vi "Estrazione Energia Detector.vi"(6 "External File?":bool, 7 "file path (dialog if empty)":path, 11 "Detector In":dbl[][](array[numeric])) -> (3 "detector-lines":T1)   [LabVIEW 2023]
uses:
  <vilib>/Utility/file.llb/Read Delimited Spreadsheet (DBL).vi
  <vilib>/gmath/NI_Gmath.lvlib
panel:
  out "Detector":dbl[][](array[numeric])
  out "Array":dbl[][](array[numeric])
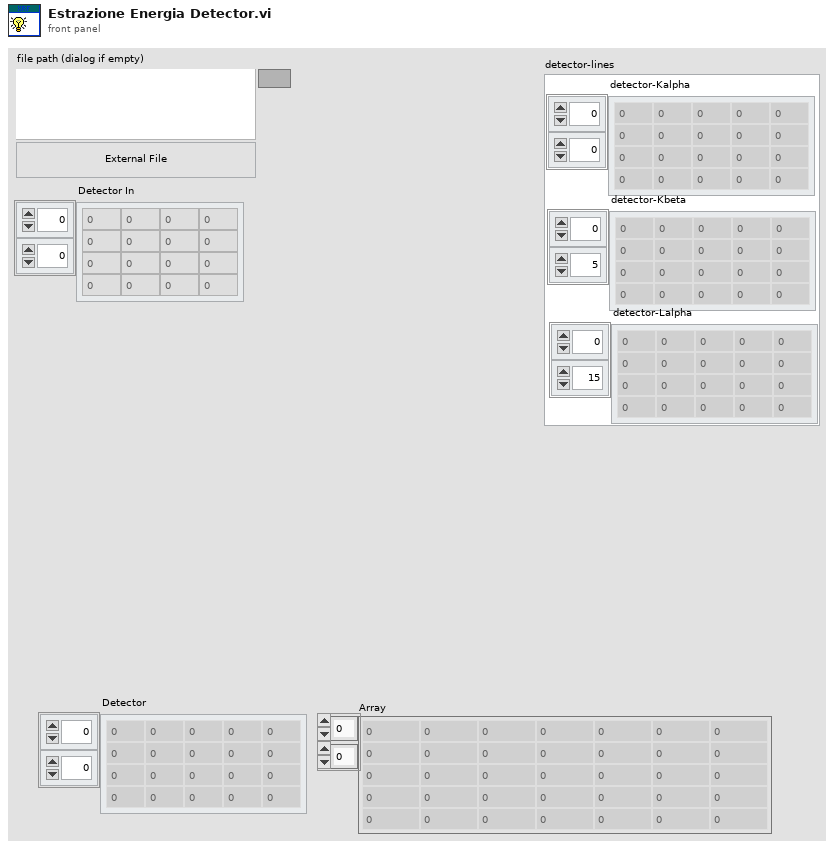
[diagram p1: front panel]
types:
  T1 = cluster{"detector-Kalpha":dbl[][], "detector-Kbeta":dbl[][], "detector-Lalpha":dbl[][]}
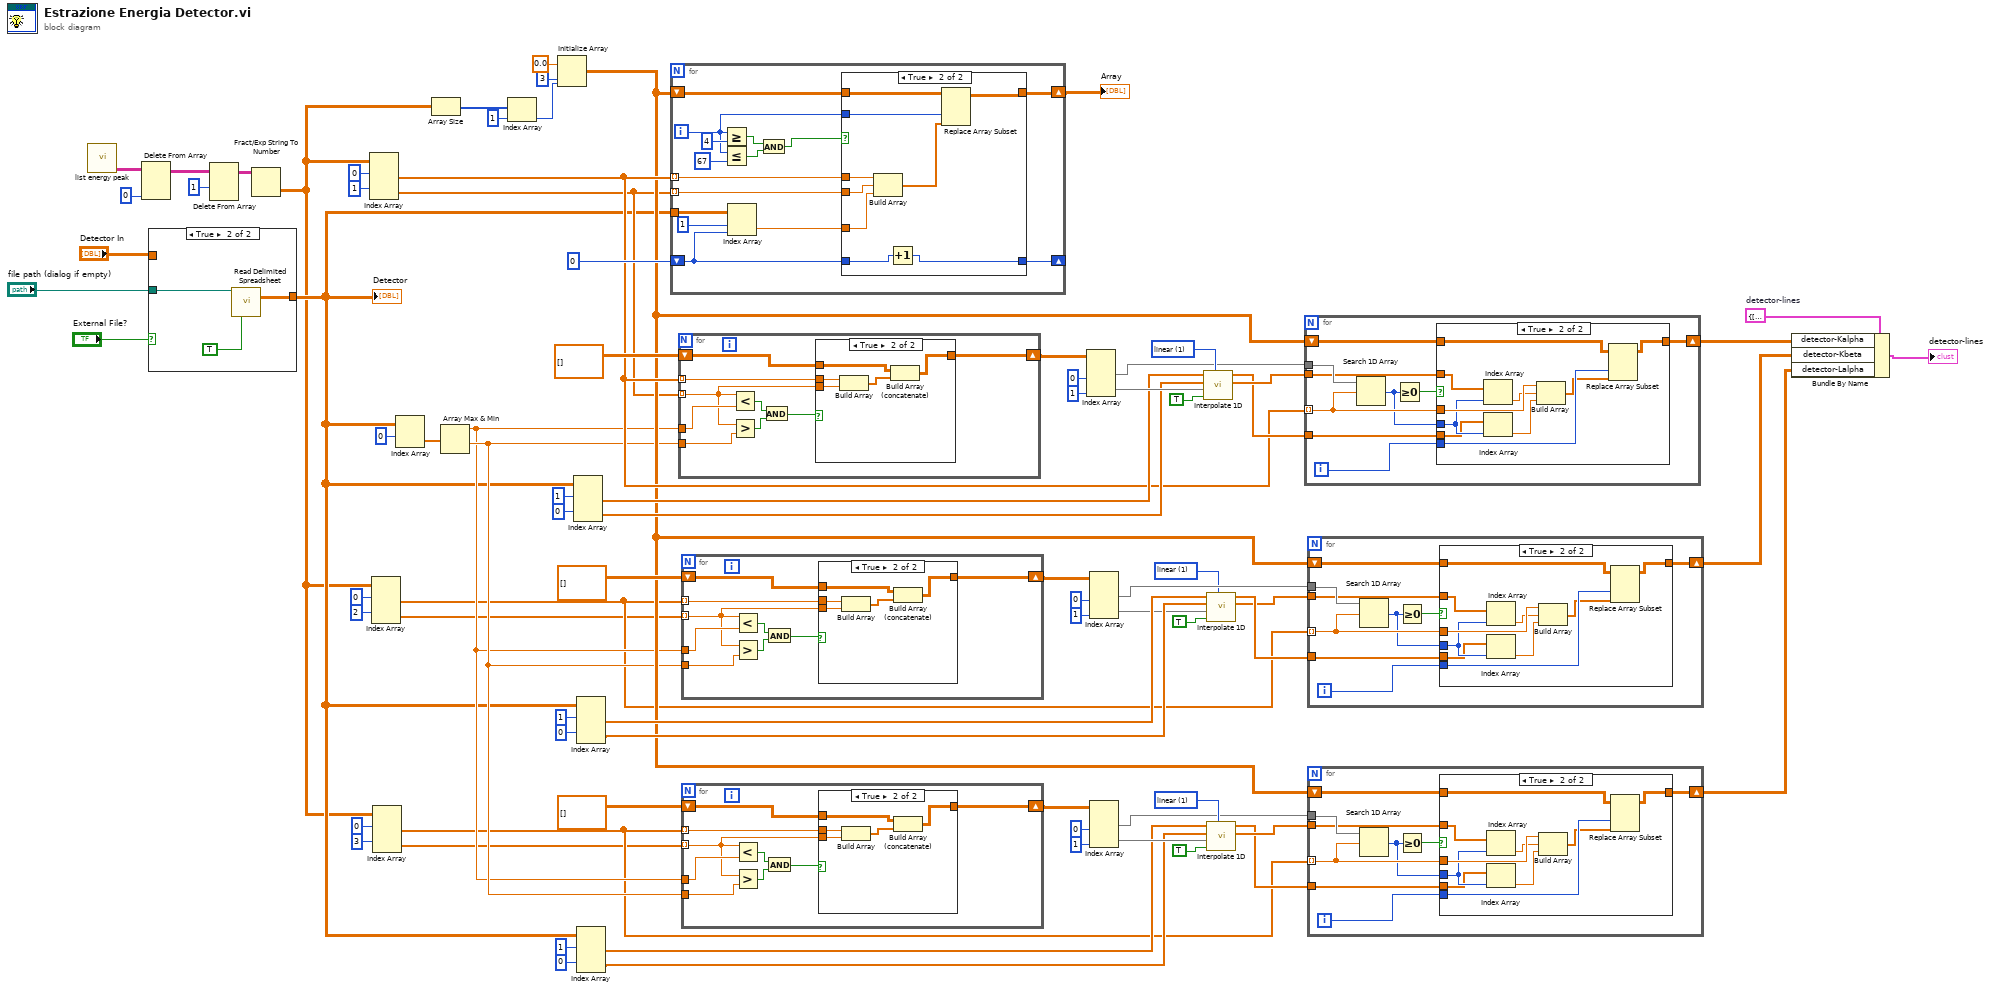
[diagram p0: block diagram]
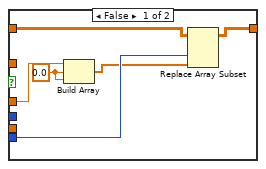
[diagram p2: hidden frame]
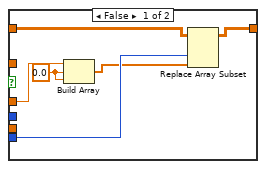
[diagram p4: hidden frame]
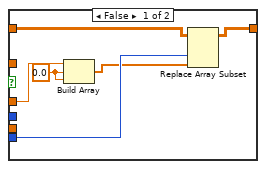
[diagram p6: hidden frame]
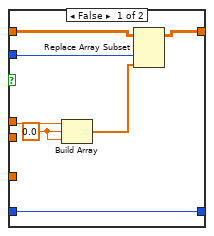
[diagram p8: hidden frame]
diagram:
  w14 = T1 {"detector-Kalpha"=[], "detector-Kbeta"=[], "detector-Lalpha"=[]}  # detector-lines
  w31 = 1 items=["nearest", "linear", "spline", "cubic Hermite", "Lagrange"] ("method")
  w40 = 1 items=["nearest", "linear", "spline", "cubic Hermite", "Lagrange"] ("method")
  w61 = 1 items=["nearest", "linear", "spline", "cubic Hermite", "Lagrange"] ("method")
  n1 = call "list energy peak.vi"() -> ("Lines"=w77:string[][])  [unwired: 6 in, 5 out]
  n2 = Delete From Array(array=w77, index (col)=0 ("disabled index (col)")) -> (array with subset deleted=w79:string[][])  [unwired: 2 in, 1 out]
  n3 = case shown="True" "External File?" {
    tunnel: [w82 w84] -> w15
    tunnel: "file path (dialog if empty)" -> [_ w83]
    tunnel: "Detector In" -> [w82 _]
    frame False {
    }
    frame True {
      n4 = call-poly <vilib>:"Read Delimited Spreadsheet.vi"("file path (dialog if empty)"=w83, "transpose? (F)"=TRUE) -> ("all rows"=w84:dbl[][])  [unwired: 8 in, 5 out]
    }
  }
  "Detector" <- w15
  n5 = Delete From Array(array=w79, index (row)=1 ("disabled index (col)")) -> (array with subset deleted=w78:string[][])  [unwired: 2 in, 1 out]
  n6 = Fract/Exp String To Number(string=w78) -> (number=w1:dbl[][])  [unwired: 3 in, 1 out]
  n7 = Index Array(array=w1, index (row) #1=0 ("index (row)"), index (row) #2=1 ("index (row)")) -> (element #1=w20:dbl[], element #2=w16:dbl[])  [unwired: 2 in]
  n8 = Index Array(array=w1, index (row) #1=0 ("index (row)"), index (row) #2=2 ("index (row)")) -> (element #1=w5:dbl[], element #2=w4:dbl[])  [unwired: 2 in]
  n9 = Index Array(array=w1, index (row) #1=0 ("index (row)"), index (row) #2=3 ("index (row)")) -> (element #1=w3:dbl[], element #2=w2:dbl[])  [unwired: 2 in]
  n10 = Index Array(array=w15, index (row)=0) -> (element=w66:dbl[])  [unwired: 1 in]
  n11 = Array Size(array=w1) -> (size(s)=w72:i32[])
  n12 = Array Max & Min(array=w66) -> (max value=w17:dbl, min value=w18:dbl)  [unwired: 2 out]
  n13 = Index Array(array=w72, index=1) -> (element=w67:i32)
  n14 = Initialize Array(0.0 ("element"), 3 ("dimension size"), w67) -> (w19:dbl[][])
  n15 = Index Array(array=w15, index (row) #1=1 ("index (row)"), index (row) #2=0 ("index (row)")) -> (element #1=w54:dbl[], element #2=w53:dbl[])  [unwired: 2 in]
  n16 = Index Array(array=w15, index (row) #1=1 ("index (row)"), index (row) #2=0 ("index (row)")) -> (element #1=w47:dbl[], element #2=w48:dbl[])  [unwired: 2 in]
  n17 = Index Array(array=w15, index (row) #1=1 ("index (row)"), index (row) #2=0 ("index (row)")) -> (element #1=w24:dbl[], element #2=w23:dbl[])  [unwired: 2 in]
  n18 = for {
    tunnel: w20 -> [w91] mode=indexing
    tunnel: w16 -> [w92] mode=indexing
    tunnel: w15 -> [w100]
    shift-right: [w90] -> w36
    shift-left: w19 -> [w89]
    shift-right: [w86] -> _
    shift-left: 0 ("index (row)") -> [w87]
    i -> [w88]
    n19 = Greater Or Equal?(x=w88, y=4) -> (x >= y?=w96:bool)
    n20 = Less Or Equal?(x=w88, y=67) -> (x <= y?=w95:bool)
    n21 = Index Array(array=w100, index (row)=1 ("disabled index (col)"), index (col)=w87) -> (element=w93:dbl)
    n22 = And(x=w96, y=w95) -> (x .and. y?=w94:bool)
    n23 = case shown="True" w94 {
      tunnel: w93 -> [_ w111]
      tunnel: w92 -> [_ w112]
      tunnel: w91 -> [w105 w113]
      tunnel: [w102 w114] -> w90
      tunnel: w89 -> [w103 w116]
      tunnel: w88 -> [w106 w115]
      tunnel: w87 -> [w101 w109]
      tunnel: [w101 w108] -> w86
      frame False {
        w104 = 0.0
        n24 = Build Array(w105, w104, w104) -> (w107:dbl[])
        n25 = Replace Array Subset(array=w103, new element=w107, index (col)=w106) -> (w102:dbl[][])  [unwired: 1 in]
      }
      frame True {
        n26 = Build Array(w113, w112, w111) -> (w110:dbl[])
        n27 = Increment(x=w109) -> (x+1=w108:i32)
        n28 = Replace Array Subset(array=w116, new element=w110, index (col)=w115) -> (w114:dbl[][])  [unwired: 1 in]
      }
    }
  }
  "Array" <- w36
  n29 = for {
    shift-right: [w117] -> w59
    shift-left: dbl[][] [] -> [w120]
    tunnel: w20 -> [w119] mode=indexing
    tunnel: w16 -> [w118] mode=indexing
    tunnel: w17 -> [w123]
    tunnel: w18 -> [w122]
    n30 = Less?(x=w118, y=w123) -> (x < y?=w125:bool)
    n31 = Greater?(x=w118, y=w122) -> (0:w124:bool)
    n32 = And(x=w125, y=w124) -> (x .and. y?=w121:bool)
    n33 = case shown="True" w121 {
      tunnel: w120 -> [w126 w127]
      tunnel: w119 -> [_ w131]
      tunnel: w118 -> [_ w130]
      tunnel: [w126 w128] -> w117
      frame False {
      }
      frame True {
        n34 = Build Array(w131, w130) -> (w129:dbl[])
        n35 = Build Array (concatenate)(w127, w129) -> (w128:dbl[][])
      }
    }
  }
  n36 = for {
    shift-right: [w132] -> w42
    shift-left: dbl[][] [] -> [w135]
    tunnel: w5 -> [w134] mode=indexing
    tunnel: w4 -> [w133] mode=indexing
    tunnel: w17 -> [w138]
    tunnel: w18 -> [w137]
    n37 = Less?(x=w133, y=w138) -> (x < y?=w140:bool)
    n38 = Greater?(x=w133, y=w137) -> (0:w139:bool)
    n39 = And(x=w140, y=w139) -> (x .and. y?=w136:bool)
    n40 = case shown="True" w136 {
      tunnel: w135 -> [w141 w142]
      tunnel: w134 -> [_ w146]
      tunnel: w133 -> [_ w145]
      tunnel: [w141 w143] -> w132
      frame False {
      }
      frame True {
        n41 = Build Array(w146, w145) -> (w144:dbl[])
        n42 = Build Array (concatenate)(w142, w144) -> (w143:dbl[][])
      }
    }
  }
  n43 = for {
    shift-right: [w147] -> w29
    shift-left: dbl[][] [] -> [w150]
    tunnel: w3 -> [w149] mode=indexing
    tunnel: w2 -> [w148] mode=indexing
    tunnel: w17 -> [w153]
    tunnel: w18 -> [w152]
    n44 = Less?(x=w148, y=w153) -> (x < y?=w155:bool)
    n45 = Greater?(x=w148, y=w152) -> (0:w154:bool)
    n46 = And(x=w155, y=w154) -> (x .and. y?=w151:bool)
    n47 = case shown="True" w151 {
      tunnel: w150 -> [w156 w157]
      tunnel: w149 -> [_ w161]
      tunnel: w148 -> [_ w160]
      tunnel: [w156 w158] -> w147
      frame False {
      }
      frame True {
        n48 = Build Array(w161, w160) -> (w159:dbl[])
        n49 = Build Array (concatenate)(w157, w159) -> (w158:dbl[][])
      }
    }
  }
  n50 = Index Array(array=w59, index (col) #1=0 ("disabled index (col)"), index (col) #2=1 ("index (col)")) -> (element #1=w58:dbl[], element #2=w60:dbl[])  [unwired: 2 in]
  n51 = Index Array(array=w42, index (col) #1=0 ("disabled index (col)"), index (col) #2=1 ("index (col)")) -> (element #1=w43:dbl[], element #2=w41:dbl[])  [unwired: 2 in]
  n52 = Index Array(array=w29, index (col) #1=0 ("disabled index (col)"), index (col) #2=1 ("index (col)")) -> (element #1=w28:dbl[], element #2=w30:dbl[])  [unwired: 2 in]
  n53 = call <vilib>:"Interpolate 1D.vi"("method"=w61, "X is monotonic"=TRUE, "xi"=w60, "X"=w53, "Y"=w54) -> ("xi used"=w57:dbl[], "yi"=w51:dbl[])  [unwired: 4 in, 1 out]
  n54 = call <vilib>:"Interpolate 1D.vi"("method"=w40, "X is monotonic"=TRUE, "xi"=w41, "X"=w48, "Y"=w47) -> ("xi used"=w44:dbl[], "yi"=w50:dbl[])  [unwired: 4 in, 1 out]
  n55 = call <vilib>:"Interpolate 1D.vi"("method"=w31, "X is monotonic"=TRUE, "xi"=w30, "X"=w23, "Y"=w24) -> ("xi used"=w27:dbl[], "yi"=w21:dbl[])  [unwired: 4 in, 1 out]
  n56 = for {
    tunnel: w57 -> [w163]
    tunnel: w58 -> [w165]
    tunnel: w20 -> [w166] mode=indexing
    shift-right: [w169] -> w13
    shift-left: w19 -> [w170]
    tunnel: w51 -> [w162]
    i -> [w168]
    n57 = Search 1D Array(1D array=w165, element=w166) -> (index of element=w164:i32)  [unwired: 1 in]
    n58 = Greater Or Equal To 0?(x=w164) -> (x >= 0?=w167:bool)
    n59 = case shown="True" w167 {
      tunnel: w170 -> [w176 w186]
      tunnel: [w175 w185] -> w169
      tunnel: w168 -> [w174 w184]
      tunnel: w166 -> [w172 w183]
      tunnel: w164 -> [_ w182]
      tunnel: w163 -> [_ w181]
      tunnel: w162 -> [_ w178]
      frame False {
        w173 = 0.0
        n60 = Build Array(w172, w173, w173) -> (w171:dbl[])
        n61 = Replace Array Subset(array=w176, new element=w171, index (col)=w174) -> (w175:dbl[][])  [unwired: 1 in]
      }
      frame True {
        n62 = Index Array(array=w181, index=w182) -> (element=w179:dbl)
        n63 = Index Array(array=w178, index=w182) -> (element=w177:dbl)
        n64 = Build Array(w183, w179, w177) -> (w180:dbl[])
        n65 = Replace Array Subset(array=w186, new element=w180, index (col)=w184) -> (w185:dbl[][])  [unwired: 1 in]
      }
    }
  }
  n66 = for {
    tunnel: w44 -> [w188]
    tunnel: w43 -> [w190]
    tunnel: w5 -> [w191] mode=indexing
    shift-right: [w194] -> w12
    shift-left: w19 -> [w195]
    tunnel: w50 -> [w187]
    i -> [w193]
    n67 = Search 1D Array(1D array=w190, element=w191) -> (index of element=w189:i32)  [unwired: 1 in]
    n68 = Greater Or Equal To 0?(x=w189) -> (x >= 0?=w192:bool)
    n69 = case shown="True" w192 {
      tunnel: w195 -> [w201 w211]
      tunnel: [w200 w210] -> w194
      tunnel: w193 -> [w199 w209]
      tunnel: w191 -> [w197 w208]
      tunnel: w189 -> [_ w207]
      tunnel: w188 -> [_ w206]
      tunnel: w187 -> [_ w203]
      frame False {
        w198 = 0.0
        n70 = Build Array(w197, w198, w198) -> (w196:dbl[])
        n71 = Replace Array Subset(array=w201, new element=w196, index (col)=w199) -> (w200:dbl[][])  [unwired: 1 in]
      }
      frame True {
        n72 = Index Array(array=w206, index=w207) -> (element=w204:dbl)
        n73 = Index Array(array=w203, index=w207) -> (element=w202:dbl)
        n74 = Build Array(w208, w204, w202) -> (w205:dbl[])
        n75 = Replace Array Subset(array=w211, new element=w205, index (col)=w209) -> (w210:dbl[][])  [unwired: 1 in]
      }
    }
  }
  n76 = for {
    tunnel: w27 -> [w213]
    tunnel: w28 -> [w215]
    tunnel: w3 -> [w216] mode=indexing
    shift-right: [w219] -> w11
    shift-left: w19 -> [w220]
    tunnel: w21 -> [w212]
    i -> [w218]
    n77 = Search 1D Array(1D array=w215, element=w216) -> (index of element=w214:i32)  [unwired: 1 in]
    n78 = Greater Or Equal To 0?(x=w214) -> (x >= 0?=w217:bool)
    n79 = case shown="True" w217 {
      tunnel: w220 -> [w226 w236]
      tunnel: [w225 w235] -> w219
      tunnel: w218 -> [w224 w234]
      tunnel: w216 -> [w222 w233]
      tunnel: w214 -> [_ w232]
      tunnel: w213 -> [_ w231]
      tunnel: w212 -> [_ w228]
      frame False {
        w223 = 0.0
        n80 = Build Array(w222, w223, w223) -> (w221:dbl[])
        n81 = Replace Array Subset(array=w226, new element=w221, index (col)=w224) -> (w225:dbl[][])  [unwired: 1 in]
      }
      frame True {
        n82 = Index Array(array=w231, index=w232) -> (element=w229:dbl)
        n83 = Index Array(array=w228, index=w232) -> (element=w227:dbl)
        n84 = Build Array(w233, w229, w227) -> (w230:dbl[])
        n85 = Replace Array Subset(array=w236, new element=w230, index (col)=w234) -> (w235:dbl[][])  [unwired: 1 in]
      }
    }
  }
  n86 = Bundle By Name(cluster=w14, "detector-Kalpha"=w13, "detector-Kbeta"=w12, "detector-Lalpha"=w11) -> (→"detector-lines":T1)
